vi "Task Construct3.vi"() -> ()   [LabVIEW 2015]
uses:
  Controls/FP Sample Container.ctl
  Controls/Freeze Button.ctl
  Controls/Scroll ONOFF.ctl
  Controls/Turbo ONOFF.ctl
panel:
  out "Drop Test":bool
  out "Boolean 2":bool
  out "Turbo ON/OFF":T1
  out "Scroll ON/OFF":T2
  out "Gauge 2":dbl(knob) scale=0.0..10.0
  in  "Help Button":bool
  in  "Storage 12":bool
  in  "Storage 11":bool
  in  "Storage 10":bool
  in  "Storage 9":bool
  in  "Storage 8":bool
  in  "Storage 7":bool
  in  "Storage 6":bool
  in  "Storage 5":bool
  in  "Storage 4":bool
  in  "Storage 3":bool
  in  "Storage 2":bool
  out "Boolean":bool
  in  "Syringe Heater":bool
  in  "Tank Blower 4":bool
  in  "Tank Blower 3":bool
  in  "Tank Blower 2":bool
  in  "Tank Blower 1":bool
  in  "Cold Bath 1 Freeze":T3
  in  "Cold Bath 2 Freeze":T3
  in  "Cold Bath 3 Freeze":T3
  in  "Cold Bath 4 Freeze":T3
  in  "Color Box":u32(colorbox)
  in  "Capillar Container":bool
  in  "Syringe Container":bool
  in  "PrepLine Container":bool
  in  "Sample Container 5":bool
  in  "Sample Container 4":bool
  in  "Sample Container 3":bool
  in  "Sample Container 2":bool
  in  "Storage Container 12":bool
  in  "Storage Container 11":bool
  in  "Storage Container 10":bool
  in  "Storage Container 9":bool
  in  "Storage Container 8":bool
  in  "Storage Container 7":bool
  in  "Storage Container 6":bool
  in  "Storage Container 5":bool
  in  "Storage Container 4":bool
  in  "Storage Container 3":bool
  in  "Storage Container 2":bool
  in  "Sample Container 1":bool
  in  "Storage 1":bool
  in  "Storage 1":bool
  in  "Storage 1":bool
  in  "Storage 1":bool
  in  "Storage 1":bool
  in  "Storage 1":bool
  in  "Storage 1":bool
  in  "Storage 1":bool
  in  "Storage 1":bool
  in  "Valve":bool
  in  "Transfer Line Container":bool
  in  "Color Box 2":u32(colorbox)
  in  "Storage Container 1 Drag Test":T4
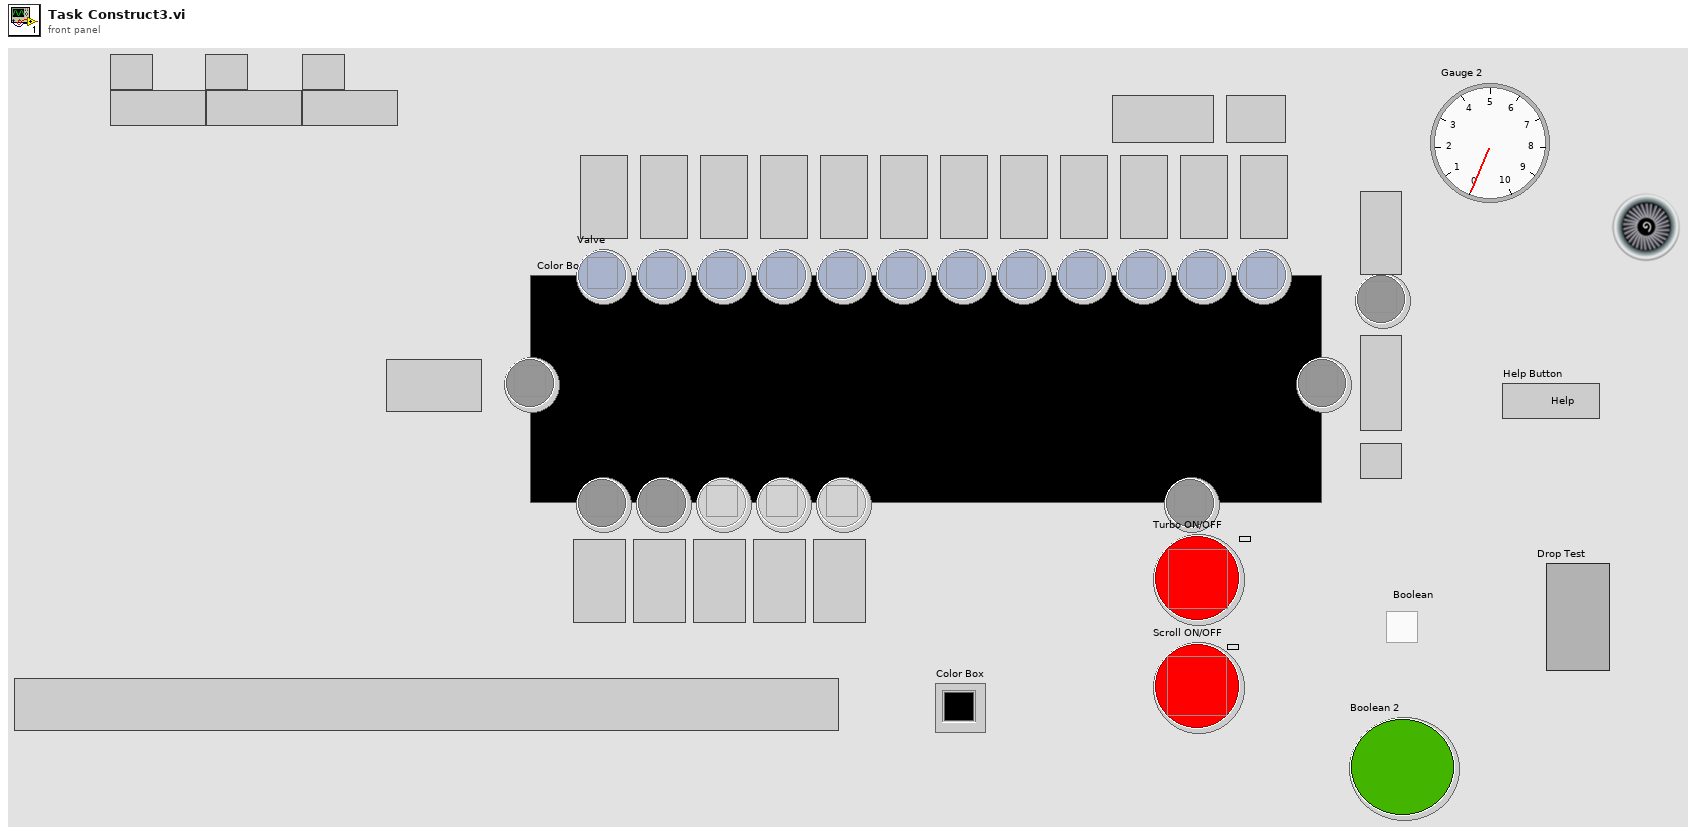
[diagram p1: front panel]
types:
  T1 = typedef "Turbo ONOFF.ctl" = bool
  T2 = typedef "Scroll ONOFF.ctl" = bool
  T3 = typedef "Freeze Button.ctl" = bool
  T4 = typedef "FP Sample Container.ctl" = bool
  T5 = cluster{"data name":string, "drag data":variant}[]
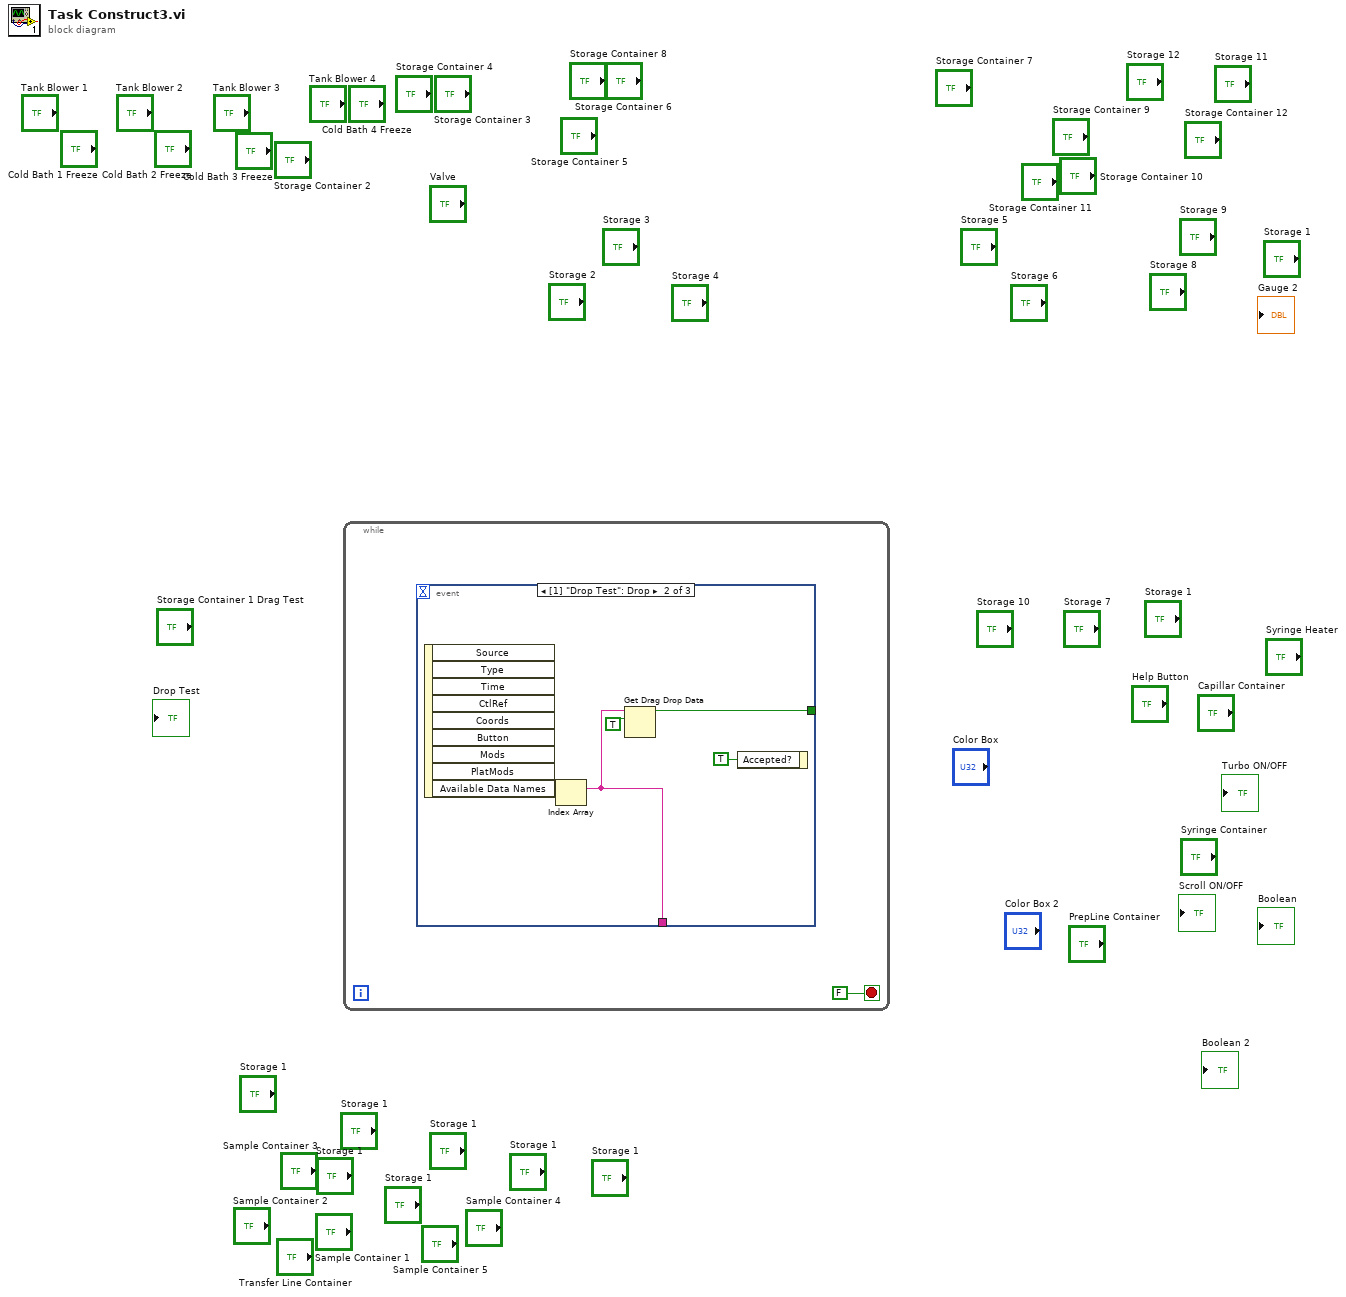
[diagram p0: block diagram]
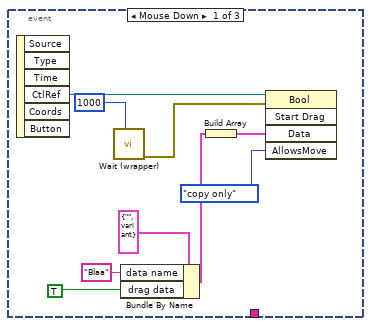
[diagram p2: hidden frame]
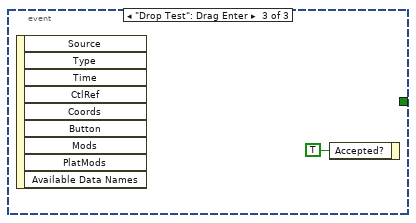
[diagram p3: hidden frame]
diagram:
  n1 = while {
    stop <- FALSE stop-if-true
    n2 = event shown="[1] \"Drop Test\": Drop" {
      selector: _ -> [_ _ _]
      dyn-events: _ -> [_ _ _]
      timeout: _ -> [_ _ _]
      tunnel: [_ w13 _] -> _
      tunnel: [_ w12 _] -> _
      event Mouse Down {
        n3 = event-data() -> ("CtlRef"=w10:refnum<vi>)  [unwired: 1 in, 5 out]
        n4 = call "Wait (wrapper).vi"("milliseconds to wait (200)"=u32 1000) -> ("error out"=w9:errorcluster)  [unwired: 10 in]
        n5 = Bundle By Name(cluster=cluster{"data name":string, "drag data":variant} {"data name"="", "drag data"=variant}, "data name"="Blaa", "drag data"=TRUE) -> (w4:cluster{"data name":string, "drag data":variant})
        n6 = Build Array(w4) -> (w3:T5)
        n7 = invoke class="Bool" method="Start Drag"(reference=w10, error in=w9, "Data"=w3, "AllowsMove"=enum32{"copy or move", "copy only", "move only"}."copy only" ("Drag Mode")) -> ()  [unwired: 1 in, 5 out]
      }
      event "Drop Test": Drop {
        n8 = event-data() -> ("Available Data Names"=w14:string[])  [unwired: 1 in, 8 out]
        n9 = Index Array(array=w14) -> (element=w13:string)  [unwired: 1 in]
        n10 = Get Drag Drop Data(8:TRUE, 9:w13) -> (3:w12:bool)  [unwired: 1 in, 1 out]
        n11 = event-data("Accepted?"=TRUE) -> ()  [unwired: 1 in, 1 out]
      }
      event "Drop Test": Drag Enter {
        n12 = event-data() -> ()  [unwired: 1 in, 9 out]
        n13 = event-data("Accepted?"=TRUE) -> ()  [unwired: 1 in, 1 out]
      }
    }
  }
